vi "emi_And Error Bool.vi"(4 "error in (no error)":errorcluster, 5 "x":bool) -> (1 "x .and. Error?":bool)   [LabVIEW 2010]
doc: "ANDs the bool and the status of teh error cluster(Error = True)"
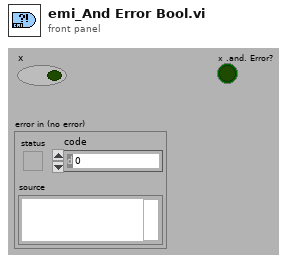
[diagram p1: front panel]
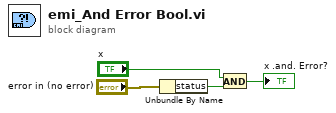
[diagram p0: block diagram]
diagram:
  n1 = Unbundle By Name("error in (no error)") -> ("status"=w2:bool)
  n2 = And(x="x", y=w2) -> (x .and. y?=→"x .and. Error?":bool)
